vi "CH_LM Initialize.vi"(0 "Address":i32=1, 1 "Serial Number":string, 3 "ID Query (True)":bool=TRUE, 4 "Reset (False)":bool, 5 "error in (no error)":errorcluster, 6 "Serial Configuration\n(19200,N,8,1)":T1={"Baud Rate"=19200, "Parity"=0, "Data Bits"=8, "Stop Bits"=1} {"Parity" items=["None", "Odd", "Even"]; "Baud Rate" items=["9600"=9600, "19200"=19200, "38400"=38400, "57600"=57600, "115200"=115200]}, 7 "Timeout / ms (3000)":i32=1000, 8 "Password":string, 9 "Lock Timeout / ms (1000)":i32=1000) -> (11 "Lock timed out":bool, 13 "timed out?":bool, 14 "Meter Index":i32, 15 "Serial Number":string, 19 "error out":errorcluster)   [LabVIEW 2012, in "CH_LM.lvlib"]
doc: "Establishes communication with the instrument and optionally performs an instrument identification query and/or an instrument reset. It also places the instrument in a default state needed for other instrument driver operations. Therefore, call this VI before calling other instrument driver VIs for this instrument. Generally, you need to call the Initialize VI only once at the beginning of an application for each meter.\n\n<B>Hint:</B> Because the Reset command will reset the realtime clock it is a password protected command that can be issued only after setting the calibration password."
uses:
  CH_LM.lvlib
  _CH_LM/CH_LM Action Enumeration.ctl
  CH_LM BaudRates.ctl
  CH_LM Parity.ctl
  CH_LM SerialConfiguration.ctl
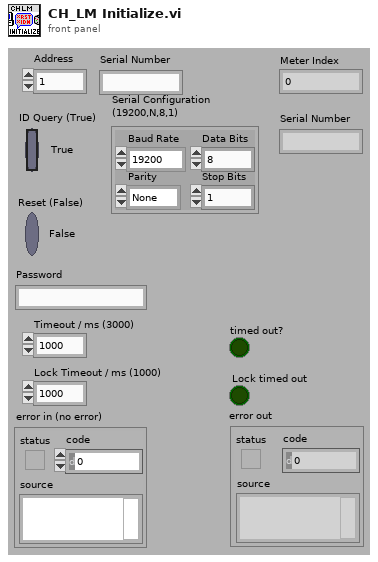
[diagram p1: front panel]
types:
  T1 = typedef "CH_LM.lvlib/CH_LM SerialConfiguration.ctl" = cluster{"Baud Rate":T2, "Parity":T3, "Data Bits":u16, "Stop Bits":u16}
  T2 = typedef "CH_LM.lvlib/CH_LM BaudRates.ctl" = u32
  T3 = typedef "CH_LM.lvlib/CH_LM Parity.ctl" = u16
  T4 = typedef "CH_LM.lvlib/CH_LM Action Enumeration.ctl" = enum16{"add", "read", "read by serial", "set", "remove", "delete", "Clear Shift-Register", ""}
  T5 = typedef "CH_LM.lvlib/CH_LM Communication Mode.ctl" = enum16{"None", "USB", "GPIB", "RS232"}
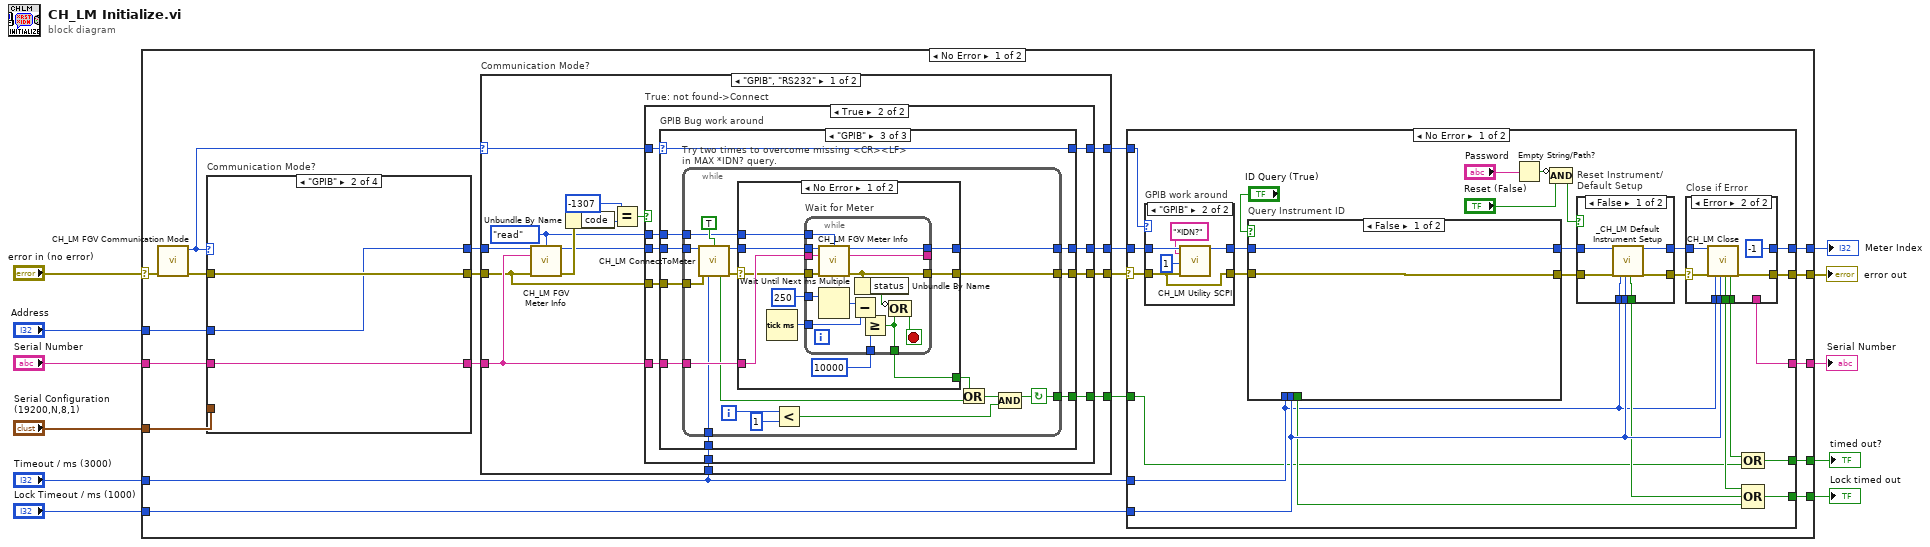
[diagram p0: block diagram]
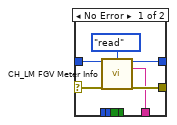
[diagram p3: hidden frame]
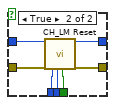
[diagram p4: hidden frame]
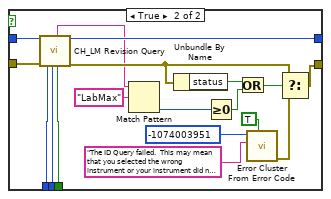
[diagram p5: hidden frame]
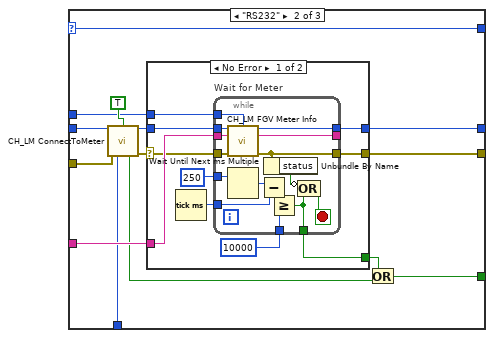
[diagram p9: hidden frame]
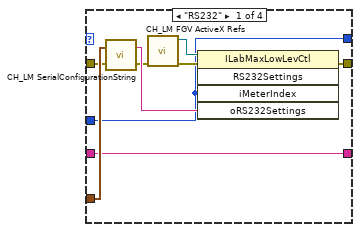
[diagram p13: hidden frame]
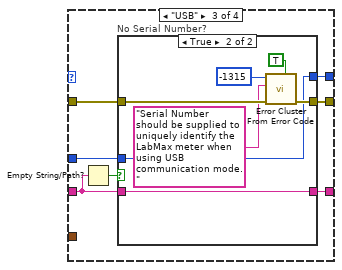
[diagram p14: hidden frame]
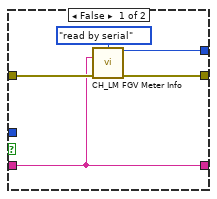
[diagram p15: hidden frame]
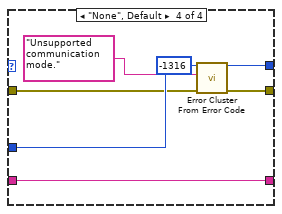
[diagram p16: hidden frame]
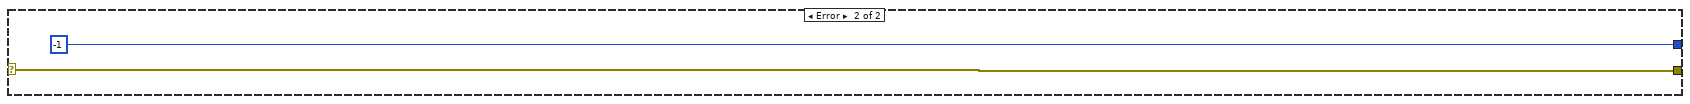
[diagram p17: hidden frame]
diagram:
  n1 = case shown="No Error" "error in (no error)" {
    selector: "error in (no error)" -> [w26 w282]
    tunnel: "Address" -> [w25 _]
    tunnel: [w31 w282] -> w11
    tunnel: [w30 -1 ("Meter Index")] -> w10
    tunnel: "Timeout / ms (3000)" -> [w14 _]
    tunnel: "Lock Timeout / ms (1000)" -> [w28 _]
    tunnel: [w29 _] -> w7
    tunnel: "Serial Number" -> [w21 _]
    tunnel: [w27 _] -> w3
    tunnel: "Serial Configuration\n(19200,N,8,1)" -> [w24 _]
    tunnel: [w13 _] -> w1
    frame No Error {
      n2 = call "CH_LM FGV Communication Mode.vi"("error in (no error)"=w26) -> ("error out"=w23:errorcluster, "Communication Mode"=w17:T5)  [unwired: 2 in, 4 out]
      n3 = case "Communication Mode?" shown="\"GPIB\"" w17 {
        tunnel: [w252 w255 w260 w277] -> w22
        tunnel: w25 -> [w245 w254 w257 w280]
        tunnel: w24 -> [w249 _ _ _]
        tunnel: w23 -> [w247 w255 w262 w278]
        tunnel: [w245 w254 w258 w280] -> w19
        tunnel: w21 -> [w244 w253 w259 w276]
        tunnel: [w244 w253 w256 w276] -> w18
        frame "RS232" {
          n4 = call "CH_LM SerialConfigurationString.vi"("error in (no error)"=w247, "Serial Configuration\n(19200,N,8,1)"=w249) -> ("error out"=w246:errorcluster, "Serial Configuration"=w248:string)
          n5 = call "CH_LM FGV ActiveX Refs.vi"("error in (no error)"=w246) -> ("error out"=w251:errorcluster, "CH_LM ActiveX Ref"=w250:refnum<k7>)  [unwired: 4 in, 2 out]
          n6 = invoke class="ILabMaxLowLevCtl" method="RS232Settings"(reference=w250, error in=w251, "iMeterIndex"=w245, "oRS232Settings"=w248) -> (error out=w252:errorcluster)  [unwired: 1 in, 4 out]
        }
        frame "GPIB" {
        }
        frame "USB" {
          n7 = Empty String/Path?(string/path=w259) -> (empty?=w261:bool)
          n8 = case "No Serial Number?" shown="True" w261 {
            tunnel: w262 -> [w267 w273]
            tunnel: [w266 w272] -> w260
            tunnel: w259 -> [w263 w270]
            tunnel: [w264 w271] -> w258
            tunnel: w257 -> [_ w271]
            tunnel: [w263 w270] -> w256
            frame False {
              n9 = call "CH_LM FGV Meter Info.vi"("Action (read)"=CH_LM_Action_Enumeration."read by serial", "Serial Number (\"\")"=w263, "error in (no error)"=w267) -> ("Meter Index out"=w264:i32, "error out"=w266:errorcluster)  [unwired: 2 in, 9 out]
            }
            frame True {
              n10 = call <vilib>:"Error Cluster From Error Code.vi"("is warning? (False)"=TRUE, "error in (no error)"=w273, "error message (\"\")"="Serial Number should be supplied to uniquely identify the LabMax meter when using USB communication mode.", "error code (0)"=-1315) -> ("error out"=w272:errorcluster)  [unwired: 1 in, 4 out]
            }
          }
        }
        frame "None", Default {
          n11 = call <vilib>:"Error Cluster From Error Code.vi"("error in (no error)"=w278, "error message (\"\")"="Unsupported communication mode.", "error code (0)"=-1316) -> ("error out"=w277:errorcluster)  [unwired: 1 in, 5 out]
        }
      }
      n12 = case "Communication Mode?" shown="\"GPIB\", \"RS232\"" w17 {
        selector: w17 -> [w117 w241]
        tunnel: w22 -> [w118 w242]
        tunnel: [w126 w243] -> w20
        tunnel: w19 -> [w127 w243]
        tunnel: w18 -> [w119 _]
        tunnel: [w123 w242] -> w15
        tunnel: [w121 _] -> w16
        tunnel: w14 -> [w120 _]
        tunnel: [w116 w241] -> w12
        frame "GPIB", "RS232" {
          w124 = CH_LM_Action_Enumeration."read" ("Action (read)")
          n13 = call "CH_LM FGV Meter Info.vi"("Meter Index"=w127, "Action (read)"=w124, "Serial Number (\"\")"=w119, "error in (no error)"=w118) -> ("Meter Index out"=w122:i32, "error out"=w128:errorcluster)  [unwired: 1 in, 9 out]
          n14 = Unbundle By Name(w128) -> ("code"=w130:i32)
          n15 = Equal?(x=-1307 ("code"), y=w130) -> (x = y?=w125:bool)
          n16 = case "True: not found->Connect" shown="True" w125 {
            tunnel: w122 -> [w133 w143]
            tunnel: [w133 w140] -> w126
            tunnel: w119 -> [_ w142]
            tunnel: w124 -> [_ w141]
            tunnel: [w132 w139] -> w123
            tunnel: [_ w137] -> w121
            tunnel: w120 -> [_ w138]
            tunnel: w118 -> [w132 w136]
            tunnel: w117 -> [w131 w135]
            tunnel: [w131 w134] -> w116
            frame False {
            }
            frame True {
              n17 = case "GPIB Bug work around" shown="\"GPIB\"" w135 {
                selector: w135 -> [w144 w147 w188]
                tunnel: w143 -> [w145 w159 w196]
                tunnel: w142 -> [_ w157 w195]
                tunnel: w141 -> [_ w156 w194]
                tunnel: [w145 w154 w193] -> w140
                tunnel: [w146 w153 w192] -> w139
                tunnel: w138 -> [_ w151 w191]
                tunnel: [_ w150 w190] -> w137
                tunnel: w136 -> [w146 w148 w189]
                tunnel: [w144 w147 w188] -> w134
                frame Default {
                }
                frame "RS232" {
                  n18 = call "CH_LM ConnectToMeter.vi"("Meter Index"=w159, "Connect?"=TRUE, "error in (no error)"=w148, "Timeout / ms (3000)"=w151) -> ("Meter Index"=w158:i32, "timed out?"=w152:bool, "error out"=w155:errorcluster)  [unwired: 9 out]
                  n19 = case shown="No Error" w155 {
                    selector: w155 -> [w164 w186]
                    tunnel: w158 -> [w167 w187]
                    tunnel: w157 -> [w166 _]
                    tunnel: w156 -> [w165 _]
                    tunnel: [w163 w187] -> w154
                    tunnel: [w162 w186] -> w153
                    tunnel: [w161 _] -> w149
                    frame No Error {
                      n20 = Tick Count (ms)() -> (millisecond timer value=w168:u32)
                      n21 = while "Wait for Meter" {
                        tunnel: [w181] -> w162
                        tunnel: w164 -> [w185]
                        tunnel: w168 -> [w182]
                        tunnel: u32 250 ("millisecond multiple") -> [w184]
                        tunnel: 10000 ("Timeout / ms (3000)") -> [w177]
                        tunnel: w166 -> [w176]
                        tunnel: [w175] -> w161
                        tunnel: [w174] -> w163
                        tunnel: [w173] -> _
                        tunnel: w165 -> [w172]
                        tunnel: w167 -> [w171]
                        stop <- w178 stop-if-true
                        n22 = call "CH_LM FGV Meter Info.vi"("Meter Index"=w171, "Action (read)"=w172, "Serial Number (\"\")"=w176, "error in (no error)"=w185) -> ("Meter Index out"=w174:i32, "Serial Number out"=w173:string, "error out"=w181:errorcluster)  [unwired: 1 in, 8 out]
                        n23 = Wait Until Next ms Multiple(millisecond multiple=w184) -> (millisecond timer value=w183:u32)
                        n24 = Subtract(x=w183, y=w182) -> (x-y=w180:u32)
                        n25 = Unbundle By Name(w181) -> ("status"=w179:bool)
                        n26 = Greater Or Equal?(x=w180, y=w177) -> (x >= y?=w175:bool)
                        n27 = Compound Arithmetic op=OR(invert w179, w175) -> (w178:bool)
                      }
                    }
                    frame Error {
                    }
                  }
                  n28 = Or(x=w149, y=w152) -> (x .or. y?=w150:bool)
                }
                frame "GPIB" {
                  n29 = while "Try two times to overcome missing <CR><LF> in MAX *IDN? query." {
                    tunnel: w196 -> [w212]
                    tunnel: w195 -> [w210]
                    tunnel: w194 -> [w209]
                    tunnel: [w207] -> w193
                    tunnel: [w206] -> w192
                    tunnel: w191 -> [w204]
                    tunnel: [w200] -> w190
                    tunnel: w189 -> [w202]
                    i -> [w199]
                    stop <- w200 continue-if-true
                    n30 = call "CH_LM ConnectToMeter.vi"("Meter Index"=w212, "Connect?"=TRUE, "error in (no error)"=w202, "Timeout / ms (3000)"=w204) -> ("Meter Index"=w211:i32, "timed out?"=w205:bool, "error out"=w208:errorcluster)  [unwired: 9 out]
                    n31 = case shown="No Error" w208 {
                      selector: w208 -> [w217 w239]
                      tunnel: w211 -> [w220 w240]
                      tunnel: w210 -> [w219 _]
                      tunnel: w209 -> [w218 _]
                      tunnel: [w216 w240] -> w207
                      tunnel: [w215 w239] -> w206
                      tunnel: [w214 _] -> w203
                      frame No Error {
                        n32 = Tick Count (ms)() -> (millisecond timer value=w221:u32)
                        n33 = while "Wait for Meter" {
                          tunnel: [w234] -> w215
                          tunnel: w217 -> [w238]
                          tunnel: w221 -> [w235]
                          tunnel: u32 250 ("millisecond multiple") -> [w237]
                          tunnel: 10000 ("Timeout / ms (3000)") -> [w230]
                          tunnel: w219 -> [w229]
                          tunnel: [w228] -> w214
                          tunnel: [w227] -> w216
                          tunnel: [w226] -> _
                          tunnel: w218 -> [w225]
                          tunnel: w220 -> [w224]
                          stop <- w231 stop-if-true
                          n34 = call "CH_LM FGV Meter Info.vi"("Meter Index"=w224, "Action (read)"=w225, "Serial Number (\"\")"=w229, "error in (no error)"=w238) -> ("Meter Index out"=w227:i32, "Serial Number out"=w226:string, "error out"=w234:errorcluster)  [unwired: 1 in, 8 out]
                          n35 = Wait Until Next ms Multiple(millisecond multiple=w237) -> (millisecond timer value=w236:u32)
                          n36 = Subtract(x=w236, y=w235) -> (x-y=w233:u32)
                          n37 = Unbundle By Name(w234) -> ("status"=w232:bool)
                          n38 = Greater Or Equal?(x=w233, y=w230) -> (x >= y?=w228:bool)
                          n39 = Compound Arithmetic op=OR(invert w232, w228) -> (w231:bool)
                        }
                      }
                      frame Error {
                      }
                    }
                    n40 = Less?(x=w199, y=1) -> (x < y?=w197:bool)
                    n41 = Or(x=w203, y=w205) -> (x .or. y?=w201:bool)
                    n42 = Compound Arithmetic op=AND(w201, w197) -> (w200:bool)
                  }
                }
              }
            }
          }
        }
        frame "USB", Default {
        }
      }
      n43 = case shown="No Error" w15 {
        selector: w15 -> [w34 w115]
        tunnel: [w57 w115] -> w31
        tunnel: [w56 w114] -> w30
        tunnel: [w55 _] -> w29
        tunnel: w28 -> [w54 _]
        tunnel: [w51 w113] -> w27
        tunnel: w14 -> [w48 _]
        tunnel: w20 -> [w36 w114]
        tunnel: w16 -> [w38 w113]
        tunnel: [w37 _] -> w13
        tunnel: w12 -> [w32 _]
        frame No Error {
          n44 = case "GPIB work around" shown="\"GPIB\"" w32 {
            tunnel: w36 -> [w59 w64]
            tunnel: [w59 w63] -> w35
            tunnel: w34 -> [w58 w60]
            tunnel: [w58 w60] -> w33
            frame "None", Default {
            }
            frame "GPIB" {
              n45 = call "CH_LM Utility SCPI.vi"("Meter Index"=w64, "SCPI Command/Query"="*IDN?", "NofStrings (-1:all)"=1, "error in (no error)"=w60) -> ("Meter Index"=w63:i32)  [unwired: 15 out]
            }
          }
          n46 = case "Query Instrument ID" shown="False" "ID Query (True)" {
            tunnel: [w93 w112] -> w46
            tunnel: [w94 w102] -> w47
            tunnel: w35 -> [w94 w101]
            tunnel: w33 -> [w93 w108]
            tunnel: w48 -> [_ w100]
            tunnel: w54 -> [_ w99]
            tunnel: [_ w98] -> w52
            frame False {
            }
            frame True {
              n47 = call "CH_LM Revision Query.vi"("Meter Index"=w101, "error in (no error)"=w108, "Timeout / ms (3000)"=w100, "Lock Timeout / ms (1000)"=w99) -> ("Module"=w95:string, "Lock timed out"=w98:bool, "Meter Index"=w102:i32, "error out"=w107:errorcluster)  [unwired: 12 out]
              n48 = Match Pattern(string=w95, regular expression="LabMax") -> (offset past match=w109:i32)  [unwired: 4 out]
              n49 = Unbundle By Name(w107) -> ("status"=w110:bool)
              n50 = Greater Or Equal To 0?(x=w109) -> (x >= 0?=w97:bool)
              n51 = Or(x=w110, y=w97) -> (x .or. y?=w111:bool)
              n52 = call <vilib>:"Error Cluster From Error Code.vi"("show call chain? (False)"=TRUE, "error message (\"\")"="The ID Query failed.  This may mean that you selected the wrong instrument or your instrument did not respond.  You may also be using a model that is not officially supported by this driver.  If you are sure that you have selected the correct instrument and it is responding, try disabling the ID Query." ("Source (VI Name)"), "error code (0)"=-1074003951 ("Code")) -> ("error out"=w103:errorcluster)  [unwired: 1 in, 5 out]
              n53 = Select(t=w107, s=w111, f=w103) -> (s? t:f=w112:errorcluster)
            }
          }
          n54 = Empty String/Path?(string/path="Password") -> (empty?=w41:bool)
          n55 = Compound Arithmetic op=AND(invert w41, "Reset (False)") -> (w39:bool)
          n56 = case "Reset Instrument/\nDefault Setup" shown="False" w39 {
            tunnel: w46 -> [w85 w91]
            tunnel: [w84 w92] -> w44
            tunnel: w47 -> [w82 w89]
            tunnel: [w83 w90] -> w45
            tunnel: w48 -> [w81 w88]
            tunnel: w54 -> [w80 w87]
            tunnel: [w79 w86] -> w53
            frame False {
              n57 = call "_CH_LM Default Instrument Setup.vi"("Meter Index"=w82, "error in (no error)"=w85, "Timeout / ms (3000)"=w81, "Lock Timeout / ms (1000)"=w80) -> ("Lock timed out"=w79:bool, "Meter Index"=w83:i32, "error out"=w84:errorcluster)  [unwired: 13 out]
            }
            frame True {
              n58 = call "CH_LM Reset.vi"("Meter Index"=w89, "error in (no error)"=w91, "Timeout / ms (3000)"=w88, "Lock Timeout / ms (1000)"=w87) -> ("Lock timed out"=w86:bool, "Meter Index"=w90:i32, "error out"=w92:errorcluster)  [unwired: 1 in, 12 out]
            }
          }
          n59 = case "Close if Error" shown="Error" w44 {
            selector: w44 -> [w68 w77]
            tunnel: w45 -> [w69 w76]
            tunnel: [w70 -1 ("Meter Index")] -> w56
            tunnel: [w67 w78] -> w57
            tunnel: w48 -> [_ w74]
            tunnel: w54 -> [_ w73]
            tunnel: [_ w72] -> w50
            tunnel: [_ w71] -> w49
            tunnel: [w65 _] -> w37
            frame No Error {
              n60 = call "CH_LM FGV Meter Info.vi"("Meter Index"=w69, "Action (read)"=CH_LM_Action_Enumeration."read", "error in (no error)"=w68) -> ("Meter Index out"=w70:i32, "Serial Number out"=w65:string, "error out"=w67:errorcluster)  [unwired: 2 in, 8 out]
            }
            frame Error {
              n61 = call "CH_LM Close.vi"("Meter Index"=w76, "error in (no error)"=w77, "Timeout / ms (3000)"=w74, "Lock Timeout / ms (1000)"=w73) -> ("Lock timed out"=w71:bool, "timed out?"=w72:bool, "error out"=w78:errorcluster)  [unwired: 13 out]
            }
          }
          n62 = Compound Arithmetic op=OR(w50, w38) -> (w51:bool)
          n63 = Compound Arithmetic op=OR(w49, w53, w52) -> (w55:bool)
        }
        frame Error {
        }
      }
    }
    frame Error {
    }
  }
  "Meter Index" <- w10
  "error out" <- w11
  "Lock timed out" <- w7
  "timed out?" <- w3
  "Serial Number" <- w1
